vi "Set ContentType.vi"(8 "error in (no error)":errorcluster, 10 "ContentType":T1="application/octet-stream", 11 "HttpHeaders_Content in":refnum<class "HttpHeaders_Content.lvclass">) -> (0 "error out":errorcluster, 3 "HttpHeaders_Content out":refnum<class "HttpHeaders_Content.lvclass">)   [LabVIEW 2018, in "HttpClient_NET.lvlib" / "HttpHeaders_Content.lvclass"]
doc: "<b> </b> <b> </b>\nHttpClient_NET\nJustin Young - Viviota\nCopyright (c) 2021\nLicense: BSD"
uses:
  HttpHeaders_Content.lvclass
  C:/Viviota/Projects/R&D/LabVIEW_HTTP_REST_NET/HTTPHeaders_NET/HttpHeaders_NET.lvclass
  Types/ContentType.ctl
  System.Net.Http
  HTTPHeaders_NET/HttpHeaders_NET.lvclass/HttpHeaders_NET.ctl
  Read NET_HttpContentHeaders.vi
  HTTPHeaders_NET/Accessors/Read NET_HttpHeaders.vi
  HttpClient_NET.lvlib
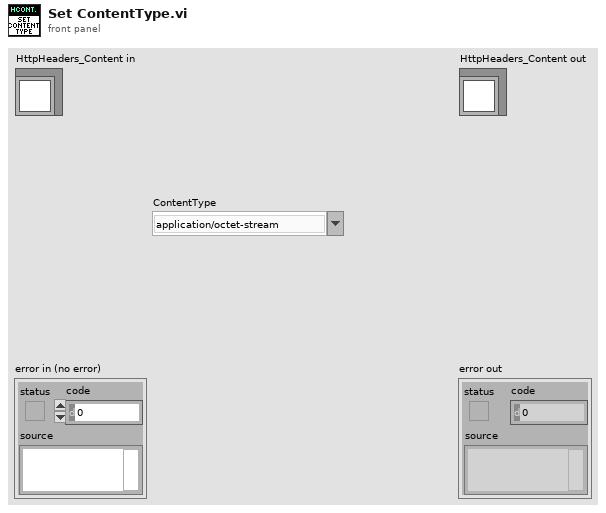
[diagram p1: front panel]
types:
  T1 = typedef "HttpClient_NET.lvlib/ContentType.ctl" = string
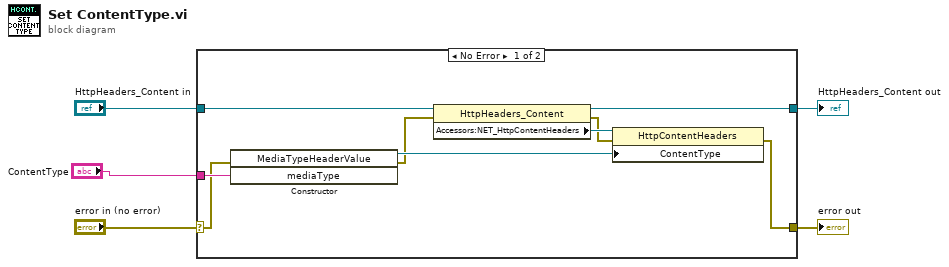
[diagram p0: block diagram]
diagram:
  n1 = case shown="No Error" "error in (no error)" {
    selector: "error in (no error)" -> [w9 w16]
    tunnel: [w6 w16] -> w4
    tunnel: [w13 w15] -> w2
    tunnel: "HttpHeaders_Content in" -> [w14 w15]
    tunnel: "ContentType" -> [w10 _]
    frame No Error {
      n2 = constructor class="MediaTypeHeaderValue"(error in=w9, "mediaType"=w10) -> (reference out=w11:refnum<k24>, error out=w8:errorcluster)  [unwired: 2 in, 2 out]
      n3 = property class="HttpHeaders_Content"(reference=w14, error in=w8) -> (reference out=w13:refnum<class "HttpHeaders_Content.lvclass">, error out=w7:errorcluster, "Accessors:NET_HttpContentHeaders"=w12:refnum<k24>)
      n4 = property class="HttpContentHeaders"(reference=w12, error in=w7, "ContentType"=w11) -> (error out=w6:errorcluster)  [unwired: 1 out]
    }
    frame Error {
    }
  }
  "error out" <- w4
  "HttpHeaders_Content out" <- w2
